vi "Identity ID.vi"(11 "ApiIdentity in":refnum<class "ApiIdentity.lvclass">) -> (2 "ID":string)   [LabVIEW 2020, in "Volatus.lvlib" / "ApiIdentity.lvclass"]
uses:
  ApiIdentity.lvclass
  ApiIdentity.lvclass/ApiIdentity.ctl
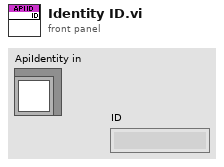
[diagram p1: front panel]
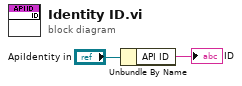
[diagram p0: block diagram]
diagram:
  n1 = Unbundle By Name("ApiIdentity in") -> ("API ID"=→"ID":string)
